vi "Initialize.vi"(8 "error in (no error)":errorcluster, 11 "DigitizerBase in":refnum<class "DigitizerBase.lvclass">) -> (0 "error out":errorcluster, 3 "DigitizerBase out":refnum<class "DigitizerBase.lvclass">)   [LabVIEW 2018, in "DigitizerPlugins.lvlib" / "DigitizerBase.lvclass"]
uses:
  DigitizerBase.lvclass
  DigitizerBase.lvclass/DigitizerBase.ctl
  Accessors/Read Handle.vi
  Accessors/Write InstRef.vi
  Accessors/Write Waveforms.vi
panel:
  in  "reset device (True)":bool=TRUE
  in  "id query (True)":bool=TRUE
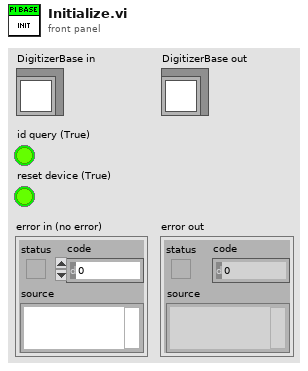
[diagram p1: front panel]
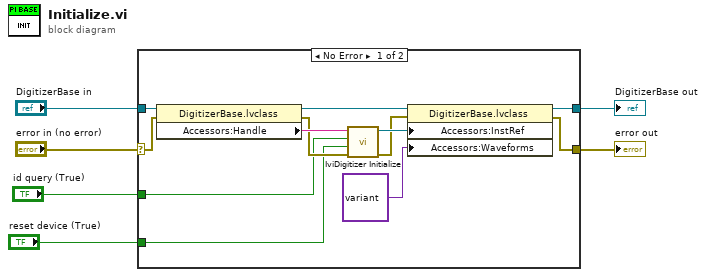
[diagram p0: block diagram]
diagram:
  n1 = case shown="No Error" "error in (no error)" {
    selector: "error in (no error)" -> [w15 w20]
    tunnel: [w8 w20] -> w5
    tunnel: [w13 w19] -> w3
    tunnel: "DigitizerBase in" -> [w18 w19]
    tunnel: "id query (True)" -> [w12 _]
    tunnel: "reset device (True)" -> [w11 _]
    frame No Error {
      n2 = property class="DigitizerBase.lvclass"(reference=w18, error in=w15) -> (reference out=w17:refnum<class "DigitizerBase.lvclass">, error out=w14:errorcluster, "Accessors:Handle"=w16:string)
      n3 = call <vilib>:"IviDigitizer Initialize.vi"("error in (no error)"=w14, "reset device (True)"=w11, "id query (True)"=w12, "logical name (SampleDigitizer)"=w16) -> ("error out"=w9:errorcluster, "instrument handle out"=w10:refnum<k15>)  [unwired: 6 in]
      n4 = property class="DigitizerBase.lvclass"(reference=w17, error in=w9, "Accessors:InstRef"=w10, "Accessors:Waveforms"=variant ("Waveforms")) -> (reference out=w13:refnum<class "DigitizerBase.lvclass">, error out=w8:errorcluster)
    }
    frame Error {
    }
  }
  "error out" <- w5
  "DigitizerBase out" <- w3
